vi "ZBX Set ATR.vi"(9 "DB 1":bool[](array[boolean])=[FALSE, FALSE, FALSE, FALSE], 11 "DB 0":bool[](array[boolean])=[FALSE, FALSE, FALSE, FALSE]) -> ()   [LabVIEW 2023]
uses:
  <vilib>/rvi/eio/common/nirviEmuTemplateMethod_errors.vi
  <vilib>/eio/EIONode/EIONode.xnode
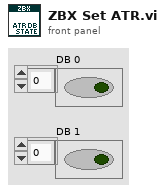
[diagram p1: front panel]
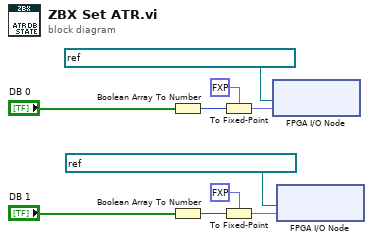
[diagram p0: block diagram]
diagram:
  n1 = Boolean Array To Number(Boolean array="DB 0") -> (number=w5:u8)
  n2 = Boolean Array To Number(Boolean array="DB 1") -> (number=w8:u8)
  n3 = To Fixed-Point(fixed-point type=fxp<+,4,4> 0.0 ("TX state"), number=w5) -> (fixed-point=w9:fxp<+,4,4>)
  n4 = To Fixed-Point(fixed-point type=fxp<+,4,4> 0.0 ("TX state"), number=w8) -> (fixed-point=w10:fxp<+,4,4>)
  n5 = xnode "FPGA I/O Node"("I/O Item"=w9, "FPGA I/O In"=refnum<k21> "Daughterboard 0\\Daughterboard State") -> ()  [unwired: 1 out]
  n6 = xnode "FPGA I/O Node"("I/O Item"=w10, "FPGA I/O In"=refnum<k21> "Daughterboard 1\\Daughterboard State") -> ()  [unwired: 1 out]
